vi "getOrigin.vi"(8 "error in (no error)":errorcluster, 11 "IDataDescriptor in":refnum<class "IDataDescriptor.lvclass">) -> (0 "error out":errorcluster, 1 "Origin":timestamp, 2 "Origin out":string, 3 "IDataDescriptor out":refnum<class "IDataDescriptor.lvclass">)   [LabVIEW 2022 SP3, in "openDAQ.lvlib" / "IBaseObject.lvlib" / "IDataDescriptor.lvlib" / "IDataDescriptor.lvclass"]
uses:
  <instrlib>/openDAQ/Public/Classes/IDataDescriptor/IDataDescriptor.lvclass
  C:/Program Files (x86)/National Instruments/LabVIEW 2022/instr.lib/openDAQ/Public/Classes/IBaseObject/IBaseObject.lvclass
  <instrlib>/openDAQ/Public/Classes/daqCoreTypes/IString/IString.lvclass
  <instrlib>/openDAQ/Public/Classes/IBaseObject/IBaseObject.lvclass/IBaseObject.ctl
  <instrlib>/openDAQ/Public/Classes/IBaseObject/Accessor/Read reference.vi
  <instrlib>/openDAQ/Public/Classes/IBaseObject/Accessor/Write reference.vi
  <instrlib>/openDAQ/Public/Classes/IDataDescriptor/IDataDescriptor.lvclass/IDataDescriptor.ctl
  <instrlib>/openDAQ/Binaries/Windows/x86/copendaq32.dll
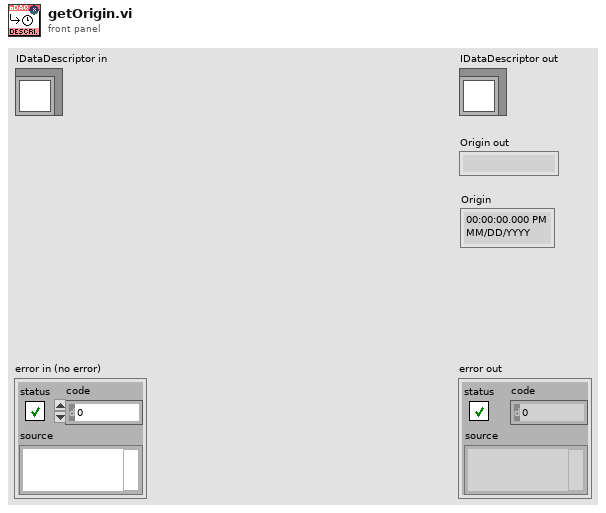
[diagram p1: front panel]
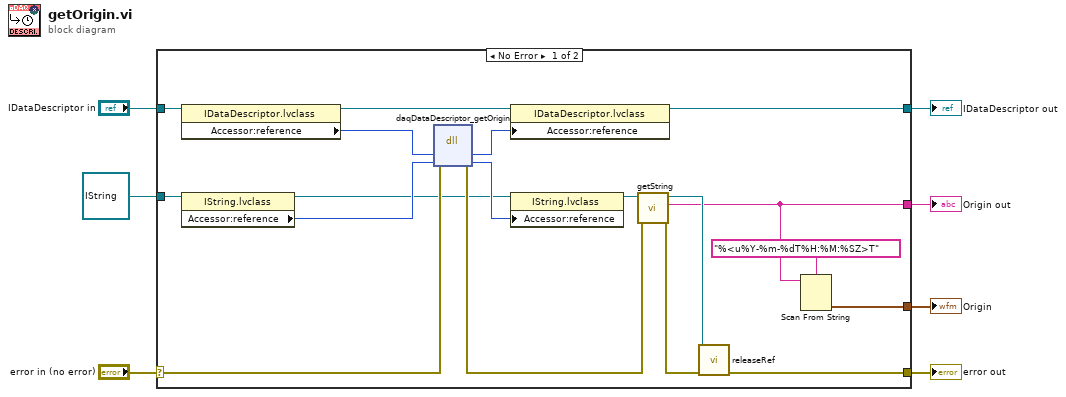
[diagram p0: block diagram]
diagram:
  n1 = case shown="No Error" "error in (no error)" {
    selector: "error in (no error)" -> [w25 w27]
    tunnel: [w12 w27] -> w6
    tunnel: [w18 w26] -> w4
    tunnel: "IDataDescriptor in" -> [w22 w26]
    tunnel: [w10 _] -> w2
    tunnel: refnum<class "IString.lvclass"> refnum ("openDAQ.lvlib:daqCoreTypes.lvlib:IString.lvclass") -> [w15 _]
    tunnel: [w8 _] -> w1
    frame No Error {
      n2 = property class="IDataDescriptor.lvclass"(reference=w22) -> (reference out=w19:refnum<class "IDataDescriptor.lvclass">, "Accessor:reference"=w21:i64)  [unwired: 1 in, 1 out]
      n3 = property class="IString.lvclass"(reference=w15) -> (reference out=w17:refnum<class "IString.lvclass">, "Accessor:reference"=w20:i64)  [unwired: 1 in, 1 out]
      n4 = dll-call lib="C:/Program Files (x86)/National Instruments/LabVIEW 2022/instr.lib/openDAQ/Binaries/Windows/x86/copendaq*.*" fn="daqDataDescriptor_getOrigin"(error in=w25, "dataDesriptior"=w21, "origin"=w20) -> (error out=w24:errorcluster, "dataDesriptior"=w16:i64, "origin"=w23:i64)  [unwired: 3 in, 1 out]
      n5 = property class="IDataDescriptor.lvclass"(reference=w19, "Accessor:reference"=w16) -> (reference out=w18:refnum<class "IDataDescriptor.lvclass">)  [unwired: 1 in, 1 out]
      n6 = property class="IString.lvclass"(reference=w17, "Accessor:reference"=w23) -> (reference out=w14:refnum<class "IString.lvclass">)  [unwired: 1 in, 1 out]
      n7 = call <instrlib>:"getString.vi"("error in (no error)"=w24, "IString in"=w14) -> ("error out"=w13:errorcluster, "String out"=w10:string, "IString out"=w11:refnum<class "IString.lvclass">)  [unwired: 7 in]
      n8 = call-dynamic "releaseRef.vi"("error in (no error)"=w13, "IBaseObject in"=w11) -> ("error out"=w12:errorcluster)  [unwired: 9 in]
      n9 = Scan From String(format string="%<u%Y-%m-%dT%H:%M:%SZ>T", input string=w10) -> (output 1=w8:timestamp)  [unwired: 3 in, 3 out]
    }
    frame Error {
    }
  }
  "error out" <- w6
  "IDataDescriptor out" <- w4
  "Origin out" <- w2
  "Origin" <- w1
